vi "Interpolation.vi"(0 "data in":T1[](array[typedef])=[{"I"=0.0, "Q"=0.0, "overflow"=FALSE}, {"I"=0.0, "Q"=0.0, "overflow"=FALSE}], 9 "input valid":bool, 11 "gen in":refnum<class "niUSRP Tx DSP v2 FPGA.lvclass">) -> (4 "data out":T1[](array[typedef]), 10 "output valid":bool, 14 "ready for input":bool, 15 "gen out":refnum<class "niUSRP Tx DSP v2 FPGA.lvclass">)   [LabVIEW 2025, in "niUSRP Tx DSP v2 FPGA.lvclass"]
uses:
  niUSRP Tx DSP v2 FPGA.lvclass
  <instrlib>/_niInstr/DSP/v1/Shared/Public/IQ Data.ctl
  niUSRP Tx DSP v2 FPGA.lvclass/niUSRP Tx DSP v2 FPGA.ctl
  <vilib>/rvi/DataTransferAndStorage/Container/Common/niFpgaContainerExecOnDevCompGetState.vi
  <vilib>/rvi/Emulation/niFpgaEmulationIsFPGAContextNoSignature.vi
  <vilib>/rvi/DataTransferAndStorage/Container/Common/niFpgaContainerGetUniqueNameForEmu.vi
  <vilib>/rvi/Memory/Memory_Emulation/niFpgaMemoryEmulationCacheClearOnFirstRun.vi
  <vilib>/rvi/Memory/Memory_Emulation/nirvimemoryEmulationManagerCache_MakeExclusive.vi
  <vilib>/rvi/Memory/Memory_Emulation/niFpgaMemoryEmulationValidateCache.vi
  <vilib>/rvi/Memory/Memory_Emulation/nirvimemoryEmulationManagerCache_InsertValue.vi
  <vilib>/Utility/error.llb/Clear Errors.vi
  <vilib>/rvi/Memory/Memory_Emulation/nirvimemoryEmulationManagerCache_ReleaseExclusive.vi
  <vilib>/rvi/Memory/Memory_Emulation/nirvimemoryEmulationManagerCache_GetValue.vi
  <vilib>/rvi/Memory/Memory_Emulation/nirvimemoryEmulationManagerCache_SetValue.vi
  <vilib>/rvi/Emulation/niFpgaProcessEmulError.vi
  <vilib>/rvi/Emulation/niFpgaSctlEmulationGetInTimedLoop.vi
  <vilib>/rvi/DataTransferAndStorage/Container/XNode/niFpgaContainer.xnode
  <vilib>/rvi/DataTransferAndStorage/Register/Emulation/niFpgaRegisterEmulationRefIn.vi
  <instrlib>/_niInstr/DSP Control/Interface/v1/FPGA/Interpolation/IQ 18-bit/Interpolation Interface (IQ 18-bit).lvclass
  <instrlib>/_niInstr/Basic Elements/v1/FPGA/niInstr Basic Elements v1 FPGA.lvlib
  <instrlib>/_niInstr/DSP/v1/Shared/niInstr DSP v1 Shared.lvlib
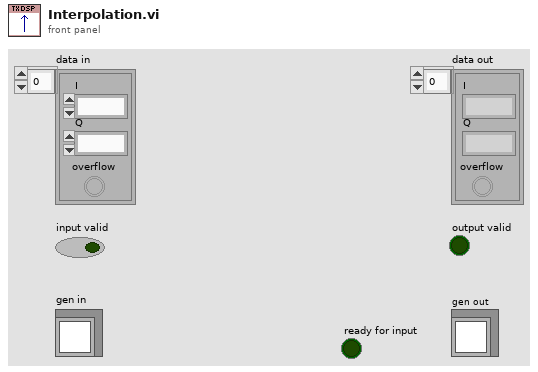
[diagram p1: front panel]
types:
  T1 = typedef "niInstr DSP v1 Shared.lvlib/IQ Data.ctl" = cluster{"I":fxp<+/-,18,1>, "Q":fxp<+/-,18,1>, "overflow":bool}
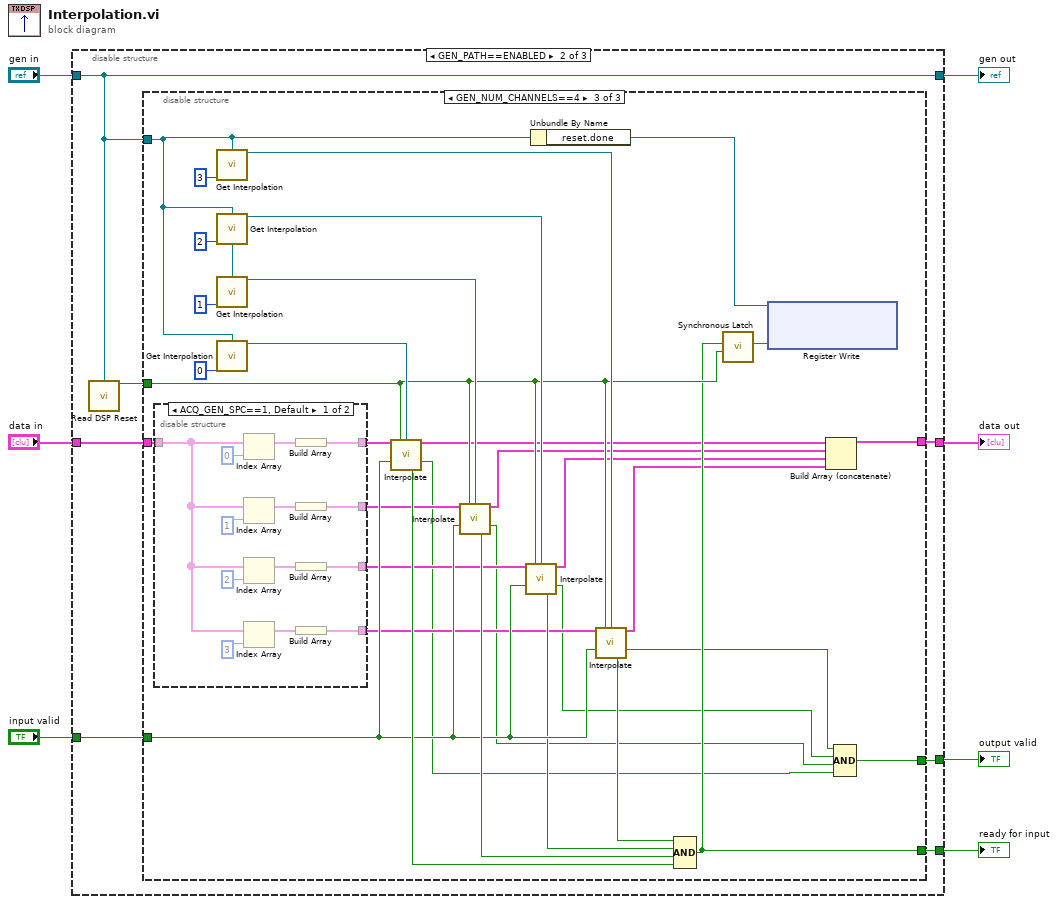
[diagram p0: block diagram]
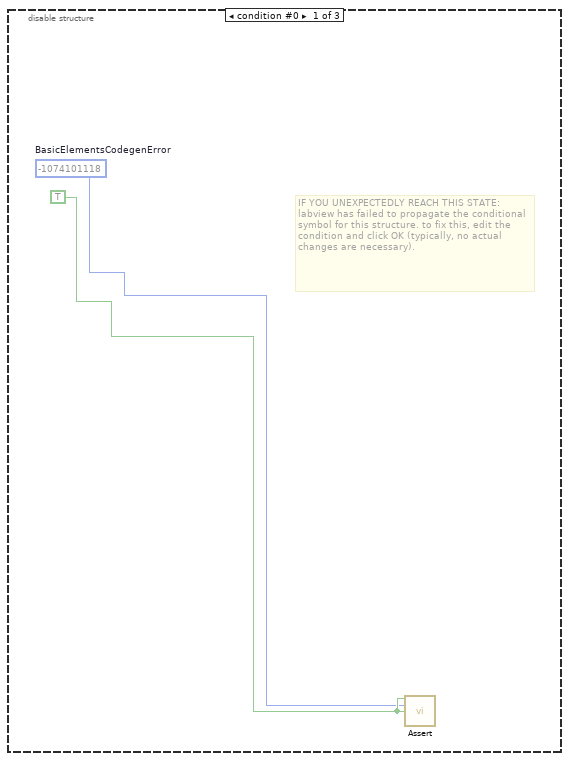
[diagram p2: hidden frame]
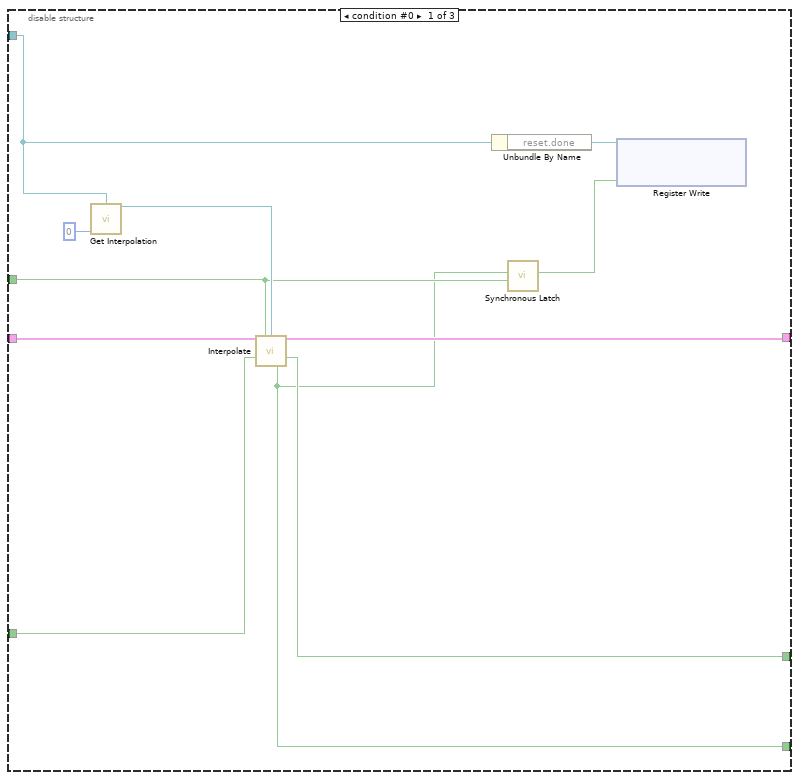
[diagram p3: hidden frame]
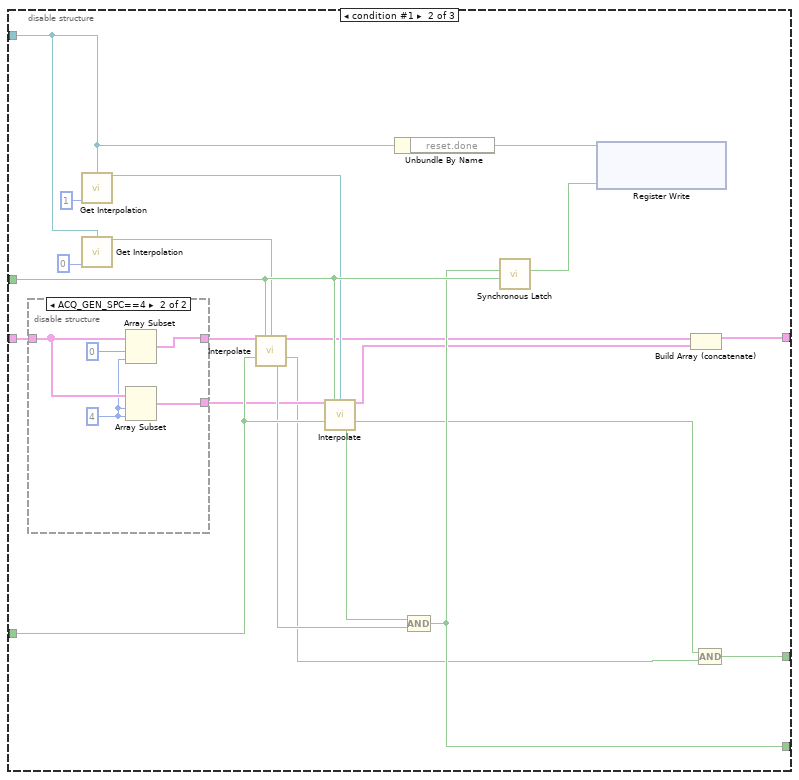
[diagram p4: hidden frame]
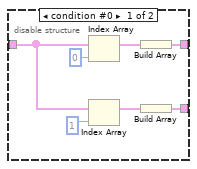
[diagram p5: hidden frame]
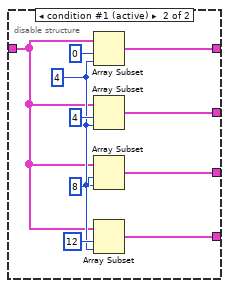
[diagram p6: hidden frame]
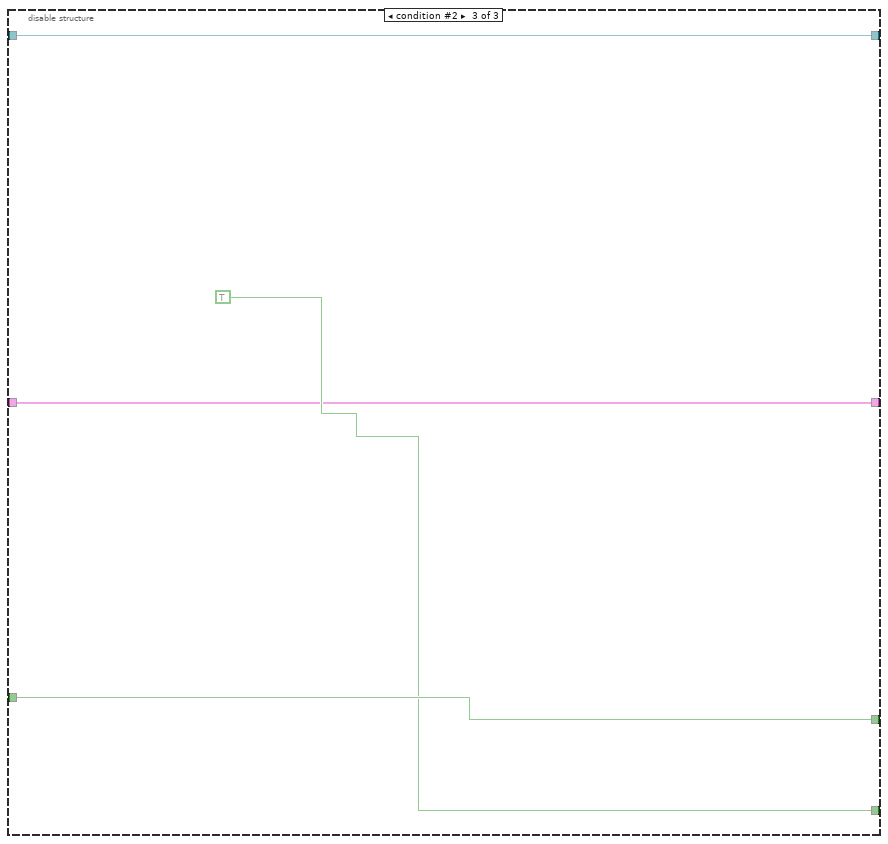
[diagram p7: hidden frame]
diagram:
  n1 = disable-structure shown="GEN_PATH==ENABLED" {
    disable-tunnel: "data in" -> [_ w15 w117]
    disable-tunnel: "input valid" -> [_ w13 w119]
    disable-tunnel: [_ w11 w119] -> w5
    disable-tunnel: [_ w10 w117] -> w4
    disable-tunnel: "gen in" -> [_ w14 w120]
    disable-tunnel: [_ w14 w120] -> w3
    disable-tunnel: [_ w12 TRUE] -> w2
    frame condition #0 {
      w9 = TRUE ("assert")
      w8 = -1074101118  # BasicElementsCodegenError
      # "IF YOU UNEXPECTEDLY REACH THIS STATE:\nlabview has failed to propagate the conditional symbol for this structure. to fix this, edit the condition and click OK (typically, no actual changes are necessary)."
      n2 = call <instrlib>:"Assert.vi"("assert"=w9, "error code"=w8, "enable show error"=w9) -> ()  [unwired: 13 in]
    }
    frame condition #1 (active) {
      n3 = call-dynamic "Read DSP Reset.vi"("gen"=w14) -> ("dsp reset"=w16:bool)  [unwired: 14 in]
      n4 = disable-structure shown="GEN_NUM_CHANNELS==4" {
        disable-tunnel: w16 -> [w24 w44 w78]
        disable-tunnel: w15 -> [w18 w35 w73]
        disable-tunnel: w14 -> [w23 w48 w81]
        disable-tunnel: w13 -> [w22 w47 w76]
        disable-tunnel: [w17 w32 w77] -> w12
        disable-tunnel: [w20 w46 w87] -> w11
        disable-tunnel: [w21 w45 w86] -> w10
        frame condition #0 {
          n5 = call-dynamic "Get Interpolation.vi"("gen"=w23, "ch"=u8 0) -> ("interpolation"=w27:refnum<class "Interpolation Interface (IQ 18-bit).lvclass">)  [unwired: 13 in]
          n6 = call-dynamic "Interpolate.vi"("data in"=w18, "reset"=w24, "interpolation"=w27, "input valid"=w22) -> ("data out"=w21:T1[], "output valid"=w20:bool, "ready for input"=w17:bool)  [unwired: 8 in, 1 out]
          n7 = Unbundle By Name(w23) -> ("reset.done"=w26:refnum<k21>)
          n8 = call <instrlib>:"Synchronous Latch.vi"("clear"=w24, "set"=w17) -> ("out"=w25:bool)  [unwired: 9 in]
          n9 = xnode ("Register Write")("Data"=w25, "Register In"=w26) -> ()  [unwired: 1 out]
        }
        frame condition #1 {
          n10 = disable-structure shown="ACQ_GEN_SPC==4" {
            disable-tunnel: w35 -> [w51 w58]
            disable-tunnel: [w50 w59] -> w33
            disable-tunnel: [w49 w57] -> w34
            frame condition #0 {
              n11 = Index Array(array=w51, index=0) -> (element=w55:T1)
              n12 = Index Array(array=w51, index=1) -> (element=w53:T1)
              n13 = Build Array(w55) -> (w50:T1[])
              n14 = Build Array(w53) -> (w49:T1[])
            }
            frame condition #1 (active) {
              w56 = 4 ("length")
              n15 = Array Subset(array=w58, index=0, length=w56) -> (w59:T1[])
              n16 = Array Subset(array=w58, index=w56, length=w56) -> (w57:T1[])
            }
          }
          n17 = call-dynamic "Get Interpolation.vi"("gen"=w48, "ch"=u8 1) -> ("interpolation"=w40:refnum<class "Interpolation Interface (IQ 18-bit).lvclass">)  [unwired: 13 in]
          n18 = call-dynamic "Get Interpolation.vi"("gen"=w48, "ch"=u8 0) -> ("interpolation"=w43:refnum<class "Interpolation Interface (IQ 18-bit).lvclass">)  [unwired: 13 in]
          n19 = call-dynamic "Interpolate.vi"("data in"=w33, "reset"=w44, "interpolation"=w43, "input valid"=w47) -> ("data out"=w31:T1[], "output valid"=w28:bool, "ready for input"=w37:bool)  [unwired: 8 in, 1 out]
          n20 = call-dynamic "Interpolate.vi"("data in"=w34, "reset"=w44, "interpolation"=w40, "input valid"=w47) -> ("data out"=w30:T1[], "output valid"=w29:bool, "ready for input"=w36:bool)  [unwired: 8 in, 1 out]
          n21 = Unbundle By Name(w48) -> ("reset.done"=w42:refnum<k21>)
          n22 = Compound Arithmetic op=AND(w36, w37) -> (w32:bool)
          n23 = call <instrlib>:"Synchronous Latch.vi"("clear"=w44, "set"=w32) -> ("out"=w41:bool)  [unwired: 9 in]
          n24 = xnode ("Register Write")("Data"=w41, "Register In"=w42) -> ()  [unwired: 1 out]
          n25 = Build Array (concatenate)(w31, w30) -> (w45:T1[])
          n26 = Compound Arithmetic op=AND(w29, w28) -> (w46:bool)
        }
        frame condition #2 (active) {
          n27 = disable-structure shown="ACQ_GEN_SPC==1, Default" {
            disable-tunnel: [w102 w110] -> w72
            disable-tunnel: [w101 w109] -> w71
            disable-tunnel: [w100 w108] -> w70
            disable-tunnel: w73 -> [w95 w111]
            disable-tunnel: [w94 w107] -> w69
            frame condition #0 {
              n28 = Index Array(array=w95, index=0) -> (element=w106:T1)
              n29 = Index Array(array=w95, index=1) -> (element=w104:T1)
              n30 = Index Array(array=w95, index=2) -> (element=w96:T1)
              n31 = Index Array(array=w95, index=3) -> (element=w98:T1)
              n32 = Build Array(w106) -> (w102:T1[])
              n33 = Build Array(w104) -> (w101:T1[])
              n34 = Build Array(w96) -> (w100:T1[])
              n35 = Build Array(w98) -> (w94:T1[])
            }
            frame condition #1 (active) {
              w112 = 4 ("length")
              n36 = Array Subset(array=w111, index=0, length=w112) -> (w110:T1[])
              n37 = Array Subset(array=w111, index=4, length=w112) -> (w109:T1[])
              n38 = Array Subset(array=w111, index=8, length=w112) -> (w108:T1[])
              n39 = Array Subset(array=w111, index=12, length=w112) -> (w107:T1[])
            }
          }
          n40 = call-dynamic "Get Interpolation.vi"("gen"=w81, "ch"=u8 3) -> ("interpolation"=w79:refnum<class "Interpolation Interface (IQ 18-bit).lvclass">)  [unwired: 13 in]
          n41 = call-dynamic "Get Interpolation.vi"("gen"=w81, "ch"=u8 2) -> ("interpolation"=w80:refnum<class "Interpolation Interface (IQ 18-bit).lvclass">)  [unwired: 13 in]
          n42 = call-dynamic "Get Interpolation.vi"("gen"=w81, "ch"=u8 1) -> ("interpolation"=w90:refnum<class "Interpolation Interface (IQ 18-bit).lvclass">)  [unwired: 13 in]
          n43 = call-dynamic "Get Interpolation.vi"("gen"=w81, "ch"=u8 0) -> ("interpolation"=w93:refnum<class "Interpolation Interface (IQ 18-bit).lvclass">)  [unwired: 13 in]
          n44 = call-dynamic "Interpolate.vi"("data in"=w72, "reset"=w78, "interpolation"=w93, "input valid"=w76) -> ("data out"=w68:T1[], "output valid"=w61:bool, "ready for input"=w88:bool)  [unwired: 8 in, 1 out]
          n45 = call-dynamic "Interpolate.vi"("data in"=w71, "reset"=w78, "interpolation"=w90, "input valid"=w76) -> ("data out"=w67:T1[], "output valid"=w62:bool, "ready for input"=w89:bool)  [unwired: 8 in, 1 out]
          n46 = call-dynamic "Interpolate.vi"("data in"=w70, "reset"=w78, "interpolation"=w80, "input valid"=w76) -> ("data out"=w66:T1[], "output valid"=w63:bool, "ready for input"=w75:bool)  [unwired: 8 in, 1 out]
          n47 = Unbundle By Name(w81) -> ("reset.done"=w92:refnum<k21>)
          n48 = call-dynamic "Interpolate.vi"("data in"=w69, "reset"=w78, "interpolation"=w79, "input valid"=w76) -> ("data out"=w65:T1[], "output valid"=w64:bool, "ready for input"=w74:bool)  [unwired: 8 in, 1 out]
          n49 = Compound Arithmetic op=AND(w74, w75, w89, w88) -> (w77:bool)
          n50 = call <instrlib>:"Synchronous Latch.vi"("clear"=w78, "set"=w77) -> ("out"=w91:bool)  [unwired: 9 in]
          n51 = xnode ("Register Write")("Data"=w91, "Register In"=w92) -> ()  [unwired: 1 out]
          n52 = Build Array (concatenate)(w68, w67, w66, w65) -> (w86:T1[])
          n53 = Compound Arithmetic op=AND(w64, w63, w62, w61) -> (w87:bool)
        }
      }
    }
    frame condition #2 {
    }
  }
  "data out" <- w4
  "output valid" <- w5
  "ready for input" <- w2
  "gen out" <- w3
